vi "Clear Data.vi"(8 "error in (no error)":errorcluster, 11 "Carya Config in":refnum<class "Carya Config.lvclass">) -> (0 "error out":errorcluster, 3 "Carya Config out":refnum<class "Carya Config.lvclass">)   [LabVIEW 2013, in "Carya Config.lvclass"]
doc: "Copyright 2018, Carya Automatisering, Wiebe Walstra."
uses:
  Carya Config.lvclass
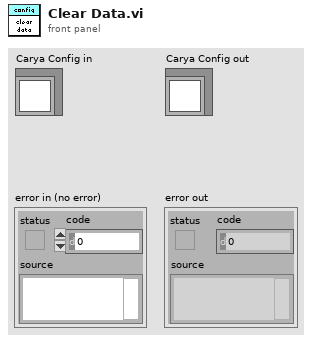
[diagram p1: front panel]
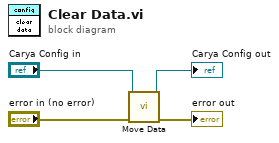
[diagram p0: block diagram]
diagram:
  n1 = call "Move Data.vi"("error in (no error)"="error in (no error)", "Carya Config dest"="Carya Config in") -> ("error out"=→"error out":errorcluster, "Carya Config out"=→"Carya Config out":refnum<class "Carya Config.lvclass">)  [unwired: 8 in]
